vi "ConfigurePWM.vi"(4 "Frequency (Hz)":dbl=100.0, 5 "Channel":i32, 6 "error in":errorcluster) -> (0 "error out":errorcluster)   [LabVIEW 2014]
doc: "Configure a channel for Pulse Width Modulation (PWM). The PWM is implemented in software and therefore limited in speed as well as subject to jitter.\n\nThe channel must be configured as an output before calling this VI."
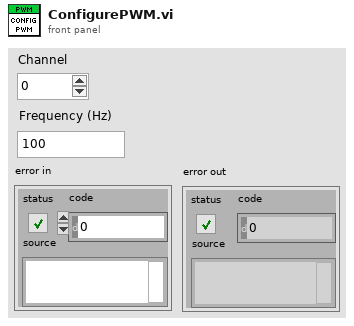
[diagram p1: front panel]
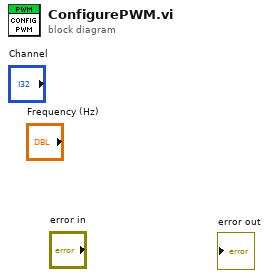
[diagram p0: block diagram]
diagram:
